vi "Create Ascii Header.vi"(8 "Log Name":string, 9 "Sys Channel Names":string[](array[string]), 10 "Step Size":dbl, 11 "Date Created":timestamp) -> (1 "Header Spreadsheet String":string, 2 "Step Size dup":dbl, 3 "Date Created dup":timestamp)   [LabVIEW 2010, in "TDMS to ASCII Convert.lvlib"]
uses:
  TDMS to ASCII Convert.lvlib
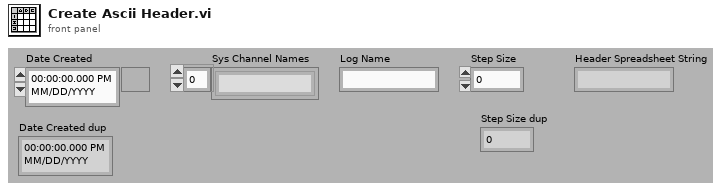
[diagram p1: front panel]
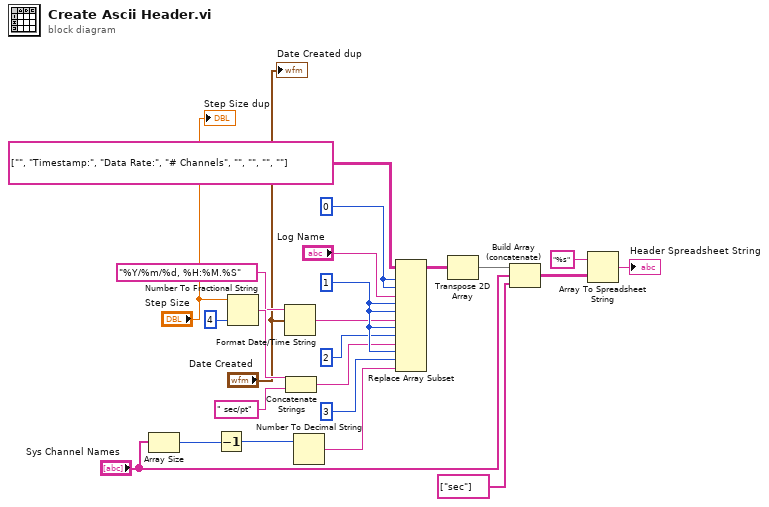
[diagram p0: block diagram]
diagram:
  w16 = 1 ("index (row)")
  w5 = 0 ("index (row)")
  n1 = Array Size(array="Sys Channel Names") -> (size(s)=w14:i32)
  n2 = Decrement(x=w14) -> (x-1=w18:i32)
  n3 = Number To Fractional String(number="Step Size", precision (6)=i16 4) -> (F-format string=w9:string)  [unwired: 2 in]
  n4 = Format Date/Time String(time format string (%c)="%Y/%m/%d, %H:%M.%S", seconds (now)="Date Created") -> (date/time string=w6:string)  [unwired: 1 in]
  n5 = Concatenate Strings(w9, " sec/pt" ("string")) -> (w11:string)
  n6 = Number To Decimal String(number=w18) -> (decimal integer string=w15:string)  [unwired: 1 in]
  n7 = Replace Array Subset(array=string[][] [["", "Timestamp:", "Data Rate:", "# Channels"], ["", "", "", ""]], new element #1="Log Name", index (row) #1=w5, index (col) #1=w5, new element #2=w6, index (row) #2=w16, index (col) #2=w16, new element #3=w11, index (row) #3=w16, index (col) #3=2 ("disabled index (col)"), new element #4=w15, index (row) #4=w16, index (col) #4=3 ("disabled index (col)")) -> (w7:string[][])
  n8 = Transpose 2D Array(2D array=w7) -> (transposed array=w19:string[][])
  n9 = Build Array (concatenate)(w19, "Sys Channel Names", string[] ["sec"] ("element")) -> (w21:string[][])
  n10 = Array To Spreadsheet String(array=w21, 3:"%s" ("format string")) -> (spreadsheet string=→"Header Spreadsheet String":string)  [unwired: 1 in]
  "Step Size dup" <- "Step Size"
  "Date Created dup" <- "Date Created"
